vi "StressControl Loop.vi"(6 "Used functions":bool, 8 "error in":errorcluster, 9 "IBM OptoElectroMechanics Configuration":T1={"Parameter Analizer"={"Parameter Analyzer VISA Session"="COM1", "Sweeping Time Parameters"={"Integration Time"=0, "Short Integration Time (s)"=1.0, "Long Integration Time (s)"=0.0, "Wait Time Parameter"=1.0}, "Acquisition Mode"=enum."Sweeping Mode", "Status Polling Time (ms)"=0, "Comment"="Test VI", "SMU 1 - Sweeping"={"Start / Offset"=0.0, "Stop / Ratio"=1.0, "Step \n(linear only)"=0.01, "Compliance"=0.1, "Power \nCompliance"=0.0, "Mode"=0, "Function"=0, "Sweep Mode"=FALSE}, "SMU 2 - Sweeping"={"Start / Offset"=0.0, "Stop / Ratio"=1.0, "Step \n(linear only)"=0.01, "Compliance"=0.1, "Power \nCompliance"=0.0, "Mode"=0, "Function"=0, "Sweep Mode"=FALSE}, "SMU 3 - Sweeping"={"Start / Offset"=0.0, "Stop / Ratio"=1.0, "Step \n(linear only)"=0.01, "Compliance"=0.1, "Power \nCompliance"=0.0, "Mode"=0, "Function"=0, "Sweep Mode"=FALSE}, "SMU 4 - Sweeping"={"Start / Offset"=0.0, "Stop / Ratio"=1.0, "Step \n(linear only)"=0.01, "Compliance"=0.1, "Power \nCompliance"=0.0, "Mode"=0, "Function"=0, "Sweep Mode"=FALSE}, "Sweep Spacing"=0, "Range"=0, "SMU1 - Sampling"={"Source"=10.0, "Compliance"=1e-05, "Mode"=0, "Function"=FALSE}, "SMU2 - Sampling"={"Source"=1.0, "Compliance"=1.0, "Mode"=0, "Function"=FALSE}, "SMU3 - Sampling"={"Source"=10.0, "Compliance"=1e-05, "Mode"=0, "Function"=FALSE}, "SMU4 - Sampling"={"Source"=0.1, "Compliance"=60.0, "Mode"=10, "Function"=FALSE}, "Sampling Time Parameters"={"Initial Interval (s)"=0.1, "Number of Samples"=60, "Total Sampling Time (s)"=10.0, "Hold Time (s)"=0.0, "Sampling Mode"=0, "Sampling Time"=0}, "Stop Condition"={"Enable Delay (s)"=0.0, "Name"="", "Threshold"=0.0, "num. of events"=1, "Event"=0, "Stop Condition Enable"=FALSE}}, "Switching Matrix"={"Switching Matrix VISA Session"="GPIB0::18::INSTR", "Connections"=[{"Connections"=[FALSE, FALSE, FALSE, FALSE, FALSE, FALSE, FALSE, FALSE, FALSE, FALSE, FALSE, FALSE], "Connection Type"=enum."Disconnected"}, {"Connections"=[FALSE, FALSE, FALSE, FALSE, FALSE, FALSE, FALSE, FALSE, FALSE, FALSE, FALSE, FALSE], "Connection Type"=enum."Disconnected"}, {"Connections"=[FALSE, FALSE, FALSE, FALSE, FALSE, FALSE, FALSE, FALSE, FALSE, FALSE, FALSE, FALSE], "Connection Type"=enum."Disconnected"}, {"Connections"=[FALSE, FALSE, FALSE, FALSE, FALSE, FALSE, FALSE, FALSE, FALSE, FALSE, FALSE, FALSE], "Connection Type"=enum."Disconnected"}, {"Connections"=[FALSE, FALSE, FALSE, FALSE, FALSE, FALSE, FALSE, FALSE, FALSE, FALSE, FALSE, FALSE], "Connection Type"=enum."Disconnected"}, {"Connections"=[FALSE, FALSE, FALSE, FALSE, FALSE, FALSE, FALSE, FALSE, FALSE, FALSE, FALSE, FALSE], "Connection Type"=enum."Disconnected"}, {"Connections"=[FALSE, FALSE, FALSE, FALSE, FALSE, FALSE, FALSE, FALSE, FALSE, FALSE, FALSE, FALSE], "Connection Type"=enum."Disconnected"}, {"Connections"=[FALSE, FALSE, FALSE, FALSE, FALSE, FALSE, FALSE, FALSE, FALSE, FALSE, FALSE, FALSE], "Connection Type"=enum."Disconnected"}]}, "Stress Control"={"Stress Control VISA Session"="StrainMotor", "Axis"=0, "Motion"=0, "Destination (°)"=0.0, "Speed (°/s)"=4.0, "Position (°)"=25.0}, "Optical Spectrometer"={"Laser Settings"={"Laser Wavelength"=enum."365 nm", "Neutral Density Filter"=enum."100%"}, "Spectrometer Settings"={"Confocal Hole Size (µm)"=0.0, "Grating"=2, "Detector"=enum."InGaAs Array"}, "Acquisition Settings"={"Acquisition Mode"=enum."Multi-Window", "Spectal Position (nm)"=632.0, "From (nm)"=735.0, "To (nm)"=0.0, "Integration Time (s)"=0.0, "Number of Accumulations"=3, "AutoScanning"=FALSE, "Spike Removal"=FALSE}, "Path"=path "C:/07 - Prizes and Awards/Marie Curie Prize/Reply Editors Final NCOMMS(10).docx"}, "Switches & Mirrors"={"Relay VISA Session"="COM1", "Switches"={"Laser"=FALSE, "Video"=FALSE}, "Delays (ms)"={"Laser"=500, "Video"=1500}}, "Camera"={"Settings"={"Pixel clock"=20, "Frame rate"=30.0, "Exposure time"=33.21525, "Master Gain"=0, "Red Gain"=0, "Green Gain"=0, "Blue Gain"=0, "Auto Gain"=FALSE, "White-balance"=FALSE, "Color Correction"=FALSE}}, "XYZ Stage"={"Connection Settings"={"Tango VISA"="", "Baudrate"=57600, "Show Protocol?"=FALSE}, "Manual Control"={"North"=FALSE, "South"=FALSE, "West"=FALSE, "East"=FALSE, "Up"=FALSE, "Down"=FALSE, "Stop"=FALSE, "XY Step"=0.0, "Z step"=0.0}, "Coordinate Control"={"Motion Mode"=enum."Absolute", "Destination [mm]"=[]}}, "AutoFocus"={"Matching Criteria"={"Minimum Score"=700.0, "Color Score Weight"=700.0, "Minimum Contrast"=50, "Match Mode"=0, "Match Feature Mode"=0, "Subpixel Accuracy"=TRUE, "Color Sensitivity"=1, "Search Strategy"=1}, "Z Scan Parameters"={"Z Range"=1380.0, "Resolution"=5000.0, "Initial Direction"=enum."Up", "Focus Threshold"=0.1, "Ascent Constant"=0.1}, "Displacement"=0.0, "Transformation Matrix"=[]}, "Sava Data"={"Workspace Info"={"Device Name"="ProberHead_Tst_C29K3_7(2)", "Device Info"="ProberHead_Tst_C29", "Path"=path "C:/Users/gio/Desktop/ProbeHeadTest"}, "Instrument Configuration"={"Instrument"=enum."Unknown Instrument", "Configuration"="Test Configuration"}, "Stress Motor Position"=0.0, "Electrical Measurement"={"Sequence"=[], "V1"=[], "V2"=[], "V3"=[], "V4"=[], "I1"=[], "I2"=[], "I3"=[], "I4"=[]}, "Optical Spectrum"={"Intensity"=[], "Wavelength"=[], "Energy"=[], "Raman Shift"=[], "Detector Temperature"=0.0}}, "PlotData"={"Sliders"={"Strain Sequence"=0, "Instrument Sequence"=0}, "Measurement"={"Which Instrument?"=enum."No Plot", "Electrical Measurement"={"Sequence"=[], "V1"=[], "V2"=[], "V3"=[], "V4"=[], "I1"=[], "I2"=[], "I3"=[], "I4"=[]}, "Measurement Mode"=enum."Sweeping Mode", "Optical Spectrum"={"Intensity"=[], "Wavelength"=[], "Energy"=[], "Raman Shift"=[], "Detector Temperature"=0.0}}, "Instrument Steps"=[], "Strain Points"=[]}, "Instrument Sequence"={"Caller VI"=enum."User"}, "Strain Measurement"={"Stress Sequence "={"Max Motor Position"=1380.0, "# Intermediate Points"=5000, "Initial Direction"=enum."Tension"}, "Track?"=FALSE}} {"AutoFocus"."Displacement" scale=1.0..1000.0; "AutoFocus"."Z Scan Parameters"."Focus Threshold" min=0.0 max=1000.0 step=1.0 format="%#_2f"; "AutoFocus"."Z Scan Parameters"."Ascent Constant" min=0.0 max=1000.0 step=1.0 format="%#_2f"; "AutoFocus"."Z Scan Parameters"."Resolution" min=0.0 max=1.0 step=0.01 format="%_2g"; "AutoFocus"."Z Scan Parameters"."Z Range" format="%_3g"; "AutoFocus"."Matching Criteria"."Match Mode" items=["Shift Invariant", "Rotation Invariant"]; "AutoFocus"."Matching Criteria"."Match Feature Mode" items=["Color and Shape", "Color", "Shape"]; "AutoFocus"."Matching Criteria"."Color Sensitivity" items=["Low Sensitivity", "Medium Sensitivity", "High Sensitivity"]; "AutoFocus"."Matching Criteria"."Search Strategy" items=["Conservative", "Balance", "Aggressive", "Very Aggressive"]; "XYZ Stage"."Manual Control"."Z step" scale=0.1..10.0; "XYZ Stage"."Manual Control"."XY Step" scale=0.1..1000.0; "Camera"."Settings"."Blue Gain" min=0 max=100 scale=0.0..100.0; "Camera"."Settings"."Green Gain" min=0 max=100 scale=0.0..100.0; "Camera"."Settings"."Red Gain" min=0 max=100 scale=0.0..100.0; "Camera"."Settings"."Master Gain" min=0 max=100 scale=0.0..100.0; "Camera"."Settings"."Exposure time" min=0.101625 max=159.246375 step=0.101625 scale=0.101625..159.246375 scale format="%#.3g"; "Camera"."Settings"."Frame rate" min=2.7455631699174137 max=6.2675785993528725 step=0.000101625 scale=2.7455631699174137..6.2675785993528725 scale format="%^#_3g"; "Camera"."Settings"."Pixel clock" min=5 max=43 scale=5.0..43.0; "PlotData"."Sliders"."Instrument Sequence" scale=0.0..10.0; "PlotData"."Sliders"."Strain Sequence" scale=0.0..10.0; "Strain Measurement"."Stress Sequence"."# Intermediate Points" max=1390; "Parameter Analizer"."Stop Condition"."Event" items=["Value > Threshold", "Value < Threshold", "| Value | > | Threshold |", "| Value | < | Threshold |"]; "Parameter Analizer"."Stop Condition"."Threshold" format="%^.2e"; "Parameter Analizer"."Stop Condition"."Enable Delay (s)" format="%.1f"; "Parameter Analizer"."Sampling Time Parameters"."Sampling Time" items=["Auto (linear only)", "No Limit", "Set Limit"]; "Parameter Analizer"."Sampling Time Parameters"."Sampling Mode" items=["Linear", "Log10", "Log25", "Log50", "Thinned Out"]; "Parameter Analizer"."Sampling Time Parameters"."Hold Time (s)" format="%.4f"; "Parameter Analizer"."Sampling Time Parameters"."Total Sampling Time (s)" format="%.1f"; "Parameter Analizer"."Sampling Time Parameters"."Initial Interval (s)" format="%^.3e"; "Parameter Analizer"."SMU 4 - Sweeping"."Function" items=["Disabled", "Var 1", "Var 2", "Var 1'", "Constant"]; "Parameter Analizer"."SMU 4 - Sweeping"."Mode" items=["V", "I", "V pulse", "I  pulse", "Common"]; "Parameter Analizer"."SMU 4 - Sweeping"."Power \nCompliance" format="%^.2e"; "Parameter Analizer"."SMU 4 - Sweeping"."Compliance" format="%^.2e"; "Parameter Analizer"."SMU 4 - Sweeping"."Step \n(linear only)" format="%^.4e"; "Parameter Analizer"."SMU 4 - Sweeping"."Stop / Ratio" format="%^.4e"; "Parameter Analizer"."SMU 4 - Sweeping"."Start / Offset" format="%^.4e"; "Parameter Analizer"."SMU 3 - Sweeping"."Function" items=["Disabled", "Var 1", "Var 2", "Var 1'", "Constant"]; "Parameter Analizer"."SMU 3 - Sweeping"."Mode" items=["V", "I", "V pulse", "I  pulse", "Common"]; "Parameter Analizer"."SMU 3 - Sweeping"."Power \nCompliance" format="%^.2e"; "Parameter Analizer"."SMU 3 - Sweeping"."Compliance" format="%^.2e"; "Parameter Analizer"."SMU 3 - Sweeping"."Step \n(linear only)" format="%^.4e"; "Parameter Analizer"."SMU 3 - Sweeping"."Stop / Ratio" format="%^.4e"; "Parameter Analizer"."SMU 3 - Sweeping"."Start / Offset" format="%^.4e"; "Parameter Analizer"."SMU 2 - Sweeping"."Function" items=["Disabled", "Var 1", "Var 2", "Var 1'", "Constant"]; "Parameter Analizer"."SMU 2 - Sweeping"."Mode" items=["V", "I", "V pulse", "I  pulse", "Common"]; "Parameter Analizer"."SMU 2 - Sweeping"."Power \nCompliance" format="%^.2e"; "Parameter Analizer"."SMU 2 - Sweeping"."Compliance" format="%^.2e"; "Parameter Analizer"."SMU 2 - Sweeping"."Step \n(linear only)" format="%^.4e"; "Parameter Analizer"."SMU 2 - Sweeping"."Stop / Ratio" format="%^.4e"; "Parameter Analizer"."SMU 2 - Sweeping"."Start / Offset" format="%^.4e"; "Parameter Analizer"."SMU 1 - Sweeping"."Function" items=["Disabled", "Var 1", "Var 2", "Var 1'", "Constant"]; "Parameter Analizer"."SMU 1 - Sweeping"."Mode" items=["V", "I", "V pulse", "I  pulse", "Common"]; "Parameter Analizer"."SMU 1 - Sweeping"."Power \nCompliance" format="%^.2e"; "Parameter Analizer"."SMU 1 - Sweeping"."Compliance" format="%^.2e"; "Parameter Analizer"."SMU 1 - Sweeping"."Step \n(linear only)" format="%^.4e"; "Parameter Analizer"."SMU 1 - Sweeping"."Stop / Ratio" format="%^.4e"; "Parameter Analizer"."SMU 1 - Sweeping"."Start / Offset" format="%^.4e"; "Parameter Analizer"."Sweeping Time Parameters"."Long Integration Time (s)" scale=0.02..2.0; "Parameter Analizer"."Sweeping Time Parameters"."Short Integration Time (s)" scale=8e-05..0.00192; "Parameter Analizer"."Sweeping Time Parameters"."Integration Time" items=["Short", "Long"]; "Parameter Analizer"."Sweeping Time Parameters"."Wait Time Parameter" format="%.1f"; "Parameter Analizer"."SMU4 - Sampling"."Mode" items=["V", "I", "Common"]; "Parameter Analizer"."SMU4 - Sampling"."Compliance" format="%^.2e"; "Parameter Analizer"."SMU4 - Sampling"."Source" format="%^.3e"; "Parameter Analizer"."SMU3 - Sampling"."Mode" items=["V", "I", "Common"]; "Parameter Analizer"."SMU3 - Sampling"."Compliance" format="%^.2e"; "Parameter Analizer"."SMU3 - Sampling"."Source" format="%^.3e"; "Parameter Analizer"."SMU2 - Sampling"."Mode" items=["V", "I", "Common"]; "Parameter Analizer"."SMU2 - Sampling"."Compliance" format="%^.2e"; "Parameter Analizer"."SMU2 - Sampling"."Source" format="%^.3e"; "Parameter Analizer"."SMU1 - Sampling"."Mode" items=["V", "I", "Common"]; "Parameter Analizer"."SMU1 - Sampling"."Compliance" format="%^.2e"; "Parameter Analizer"."SMU1 - Sampling"."Source" format="%^.3e"; "Parameter Analizer"."Range" items=["auto", "fixed", "limited"]; "Parameter Analizer"."Sweep Spacing" items=["linear", "log 10", "log 25", "log 50"]; "Stress Control"."Axis" min=1 max=3; "Stress Control"."Position (°)" format="%.6g"; "Stress Control"."Speed (°/s)" min=0.0 max=4.0 format="%.6f"; "Stress Control"."Destination (°)" min=-2000000000.0 max=2000000000.0 format="%.6f"; "Stress Control"."Motion" items=["Absolute", "Relative"]; "Optical Spectrometer"."Spectrometer Settings"."Grating" items=["1800 l/mm", "150 l/mm"]}, 10 "Message Queues out":T57, 11 "Notifiers":T44) -> (0 "error out":errorcluster)   [LabVIEW 2014]
uses:
  support/Message Queue/All Message Queues.ctl
  support/Message Queue/Message Cluster.ctl
  support/Notifiers/Notifiers.ctl
  support/Message Handler Loop Notifiers.ctl
  Hardware Control/Parameter Analyzer/Parameter Analyzer Notifiers.ctl
  Hardware Control/Switching Matrix/Switching Matrix Notifiers.ctl
  Hardware Control/Stress Control/StressControl Notifiers.ctl
  Hardware Control/Spectrometer/Spectrometer Notifiers.ctl
  Hardware Control/Switches and Mirrors/SwitchesMirrors Notifiers.ctl
  Hardware Control/Camera/Camera Notifiers.ctl
  Hardware Control/XYZ Stage/XYZ Notifications.ctl
  Hardware Control/Autofocus/Autofocus Notifiers.ctl
  Measurements/Optoelectronic Measurement/Optoelectronic Notifiers.ctl
  Measurements/Save Data/SaveData Notifiers.ctl
  Measurements/Instrument Sequence/Instrument Sequence Notifiers.ctl
  support/Configuration/Configuration.ctl
  Hardware Control/Parameter Analyzer/Parameter Analyzer Config.ctl
  Hardware Control/Parameter Analyzer/Parameter Analyzer Integration Parameters.ctl
  Hardware Control/Parameter Analyzer/Parameter Analyzer SMU Sweeping.ctl
  Hardware Control/Parameter Analyzer/Parameter Analyzer Sweep Spacing.ctl
  Hardware Control/Parameter Analyzer/Parameter Analyzer SMU Range.ctl
  Hardware Control/Parameter Analyzer/Parameter Analyzer SMU Sampling.ctl
  Hardware Control/Parameter Analyzer/Parameter Analyzer Sampling Parameters.ctl
  Hardware Control/Parameter Analyzer/Parameter Analyzer Stop Sampling Conditions.ctl
  Hardware Control/Switching Matrix/Switching Matrix Config.ctl
  Hardware Control/Stress Control/StressControl Config.ctl
  Hardware Control/Spectrometer/Spectrometer Config.ctl
  Hardware Control/Spectrometer/Laser Settings.ctl
  Hardware Control/Spectrometer/Laser.ctl
  Hardware Control/Spectrometer/Filter.ctl
  Hardware Control/Spectrometer/Grating Detector Settings.ctl
  Hardware Control/Spectrometer/Grating.ctl
  Hardware Control/Spectrometer/Detector.ctl
  Hardware Control/Spectrometer/Acquisition Settings.ctl
  Hardware Control/Switches and Mirrors/SwitchesMirrors Config.ctl
  Hardware Control/Switches and Mirrors/SwitchesMirrors Status.ctl
  Hardware Control/Camera/Camera Config.ctl
  Hardware Control/Camera/Camera Settings.ctl
  Hardware Control/XYZ Stage/XYZ Config.ctl
  Hardware Control/XYZ Stage/XYZ Connection Settings.ctl
  Hardware Control/XYZ Stage/XYZ Stage Control.ctl
  Hardware Control/XYZ Stage/XYZ Coordinate Control.ctl
  Hardware Control/Autofocus/AutoFocus Config.ctl
  Hardware Control/Autofocus/ZScan.ctl
  <vilib>/Analysis/Matrix/Datatypes/RealMatrix.ctl
  Measurements/Save Data/SaveData Config.ctl
  Measurements/Save Data/SaveData Workspace Info.ctl
  Measurements/Save Data/SaveData Instrument Configuration.ctl
  Measurements/Instrument Sequence/Instrument List.ctl
  Hardware Control/Spectrometer/Spectral Data.ctl
  Measurements/Plot Data/PlotData Config.ctl
  Measurements/Plot Data/Measurement.ctl
  Measurements/Plot Data/WhichInstrument.ctl
  Hardware Control/Parameter Analyzer/Electrical Data.ctl
  Measurements/Instrument Sequence/Instrument Steps.ctl
  Measurements/Instrument Sequence/Action.ctl
  Measurements/Instrument Sequence/Instrument Sequence Config.ctl
  Measurements/Strain Measurement/Strain Measurement Config.ctl
  Hardware Control/Stress Control/StressControl Functions.ctl
  support/Message Queue/Message Queue.lvlib
  <vilib>/Analysis/Matrix/NI_Matrix.lvlib
panel:
  # "LICENSED MATERIALS – PROPERTY OF IBM\nCopyright IBM Corp. 2016,\nALL RIGHTS RESERVED"
  # "XY"
  # "Z"
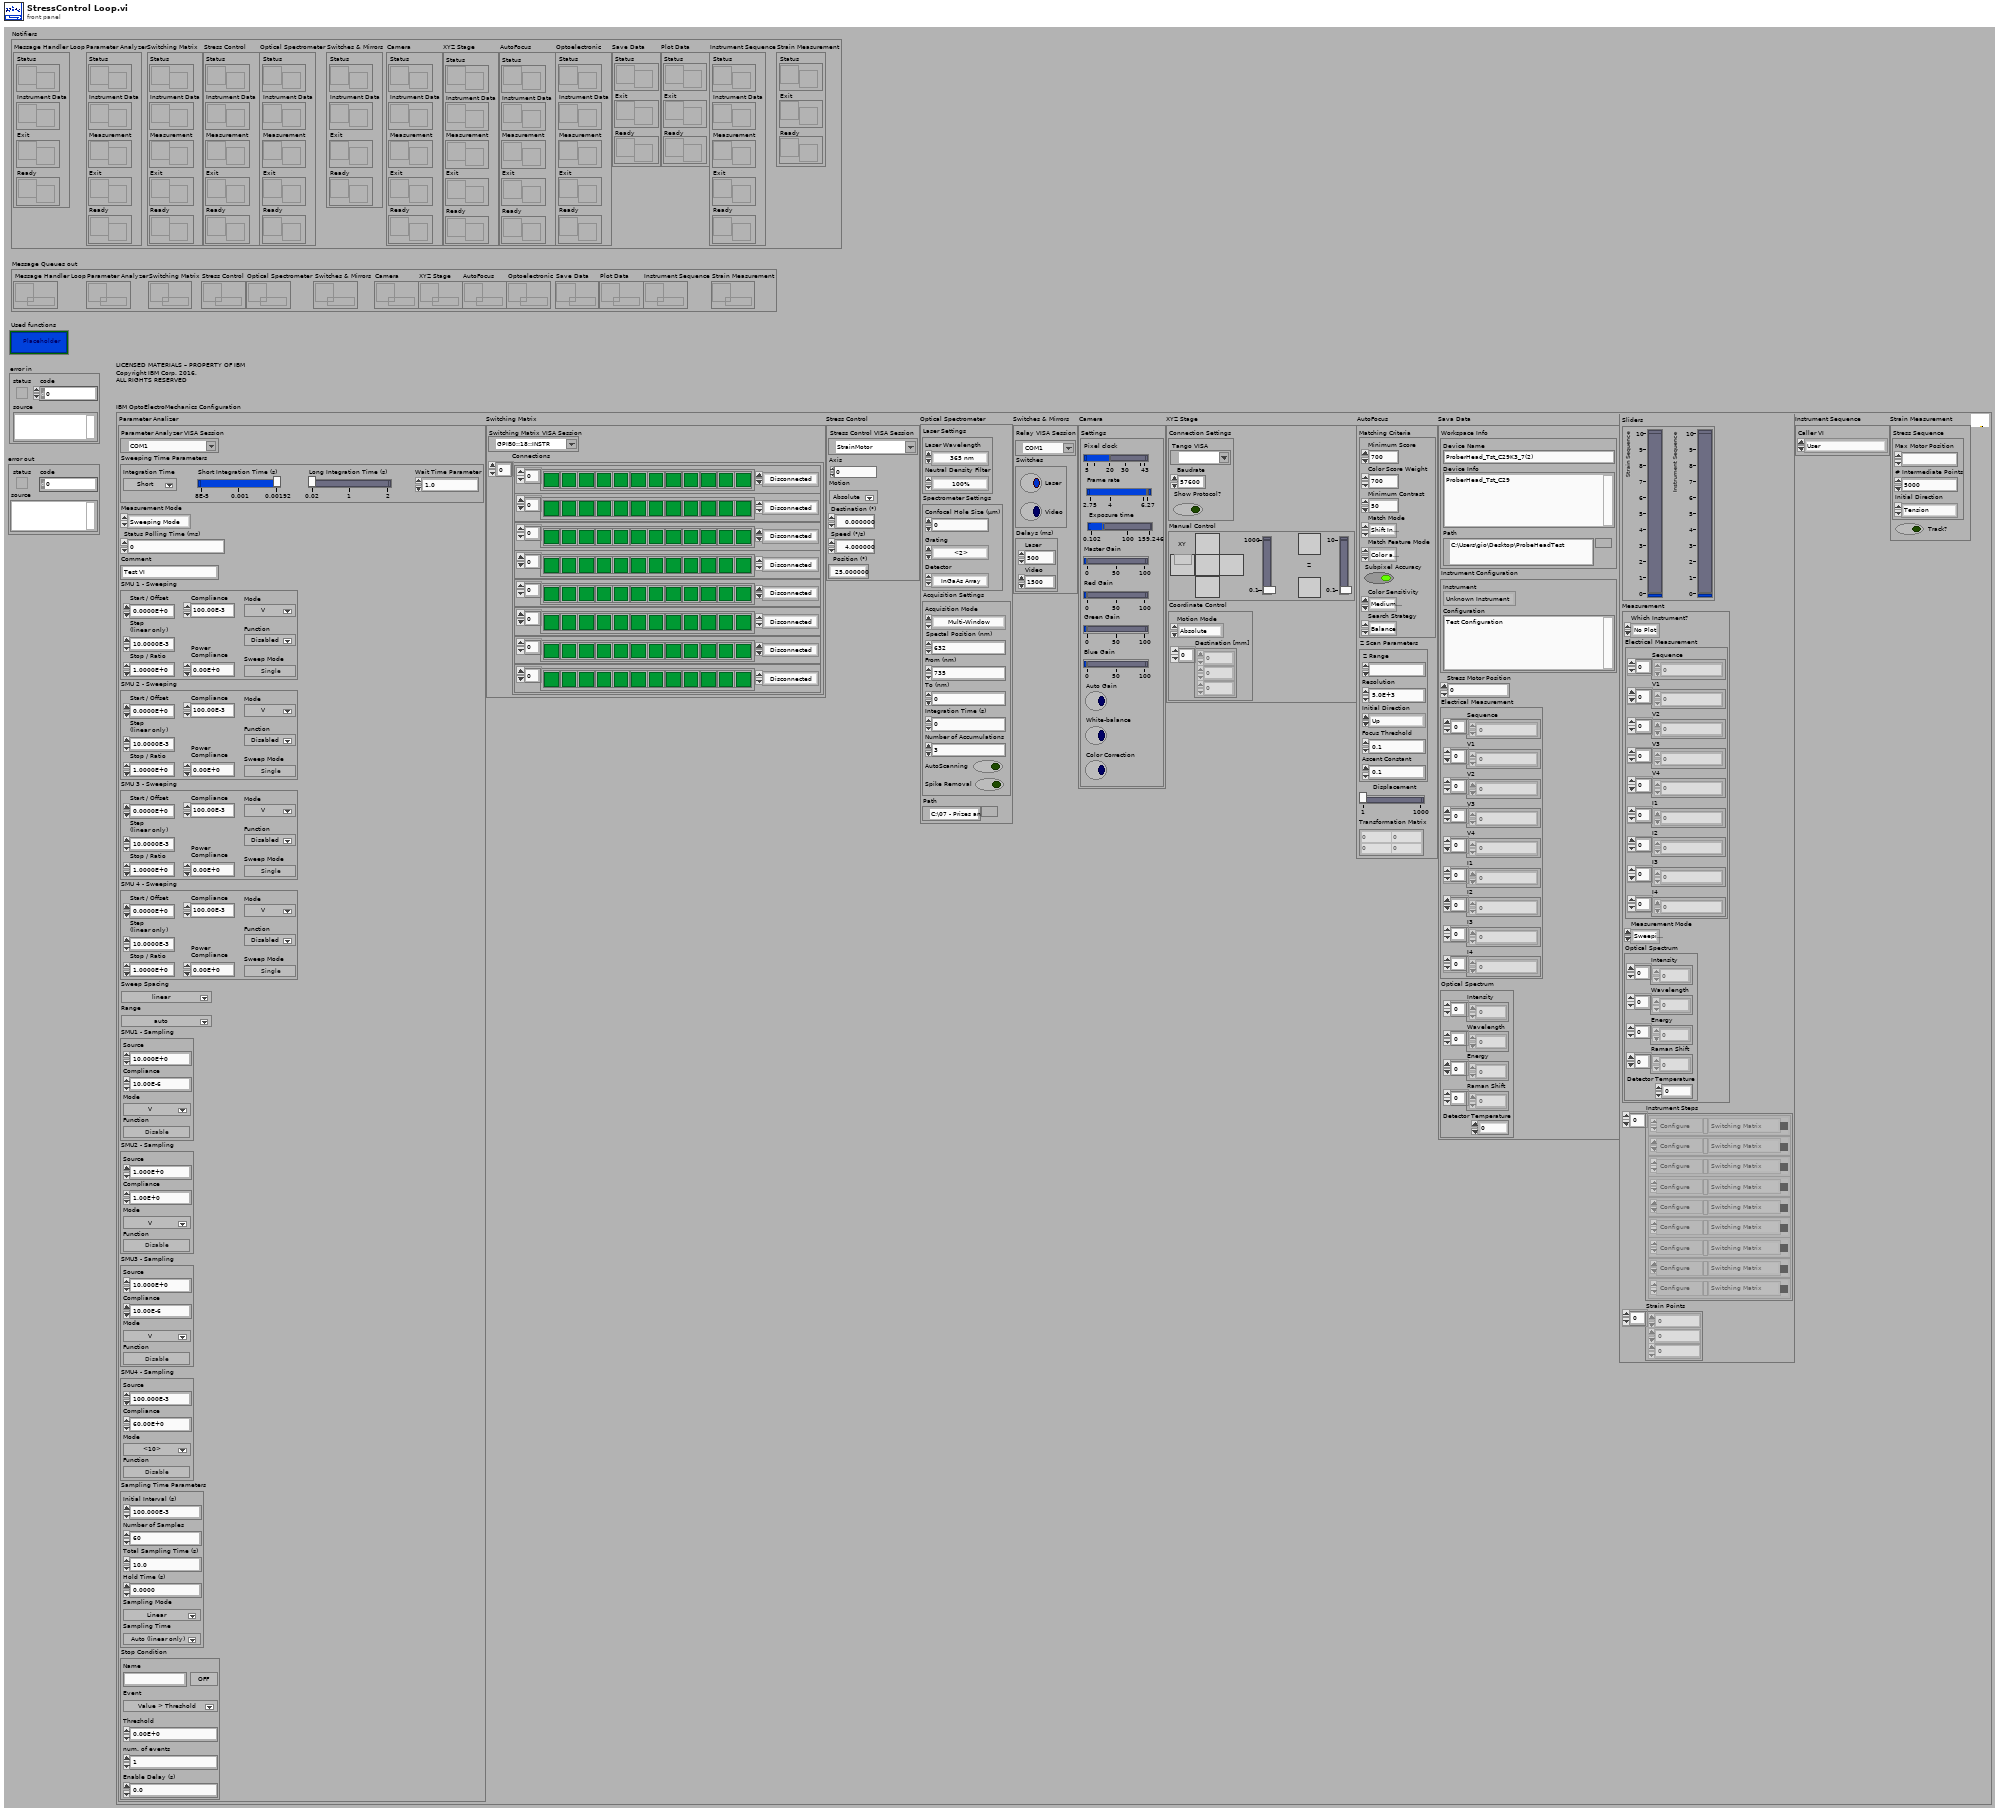
[diagram p1: front panel]
types:
  T1 = typedef "Configuration.ctl" = cluster{"Parameter Analizer":T2, "Switching Matrix":T10, "Stress Control":T11, "Optical Spectrometer":T12, "Switches & Mirrors":T20, "Camera":T22, "XYZ Stage":T24, "AutoFocus":T28, "Sava Data":T31, "PlotData":T36, "Instrument Sequence":T42, "Strain Measurement":T43}
  T2 = typedef "Parameter Analyzer Config.ctl" = cluster{"Parameter Analyzer VISA Session":refnum<visa-resource-name>, "Sweeping Time Parameters":T3, "Acquisition Mode":enum32{"Sweeping Mode", "Sampling Mode"}, "Status Polling Time (ms)":u32, "Comment":string, "SMU 1 - Sweeping":T4, "SMU 2 - Sweeping":T4, "SMU 3 - Sweeping":T4, "SMU 4 - Sweeping":T4, "Sweep Spacing":T5, "Range":T6, "SMU1 - Sampling":T7, "SMU2 - Sampling":T7, "SMU3 - Sampling":T7, "SMU4 - Sampling":T7, "Sampling Time Parameters":T8, "Stop Condition":T9}
  T3 = typedef "Parameter Analyzer Integration Parameters.ctl" = cluster{"Integration Time":u32, "Short Integration Time (s)":dbl, "Long Integration Time (s)":dbl, "Wait Time Parameter":dbl}
  T4 = typedef "Parameter Analyzer SMU Sweeping.ctl" = cluster{"Start / Offset":dbl, "Stop / Ratio":dbl, "Step \n(linear only)":dbl, "Compliance":dbl, "Power \nCompliance":dbl, "Mode":u32, "Function":i32, "Sweep Mode":bool}
  T5 = typedef "Parameter Analyzer Sweep Spacing.ctl" = u16
  T6 = typedef "Parameter Analyzer SMU Range.ctl" = u16
  T7 = typedef "Parameter Analyzer SMU Sampling.ctl" = cluster{"Source":dbl, "Compliance":dbl, "Mode":u32, "Function":bool}
  T8 = typedef "Parameter Analyzer Sampling Parameters.ctl" = cluster{"Initial Interval (s)":dbl, "Number of Samples":i32, "Total Sampling Time (s)":dbl, "Hold Time (s)":dbl, "Sampling Mode":i32, "Sampling Time":i32}
  T9 = typedef "Parameter Analyzer Stop Sampling Conditions.ctl" = cluster{"Enable Delay (s)":dbl, "Name":string, "Threshold":dbl, "num. of events":i32, "Event":i32, "Stop Condition Enable":bool}
  T10 = typedef "Switching Matrix Config.ctl" = cluster{"Switching Matrix VISA Session":refnum<visa-resource-name>, "Connections":cluster{"Connections":bool[], "Connection Type":enum16{"Disconnected", "Make - Break", "Break - Make"}}[]}
  T11 = typedef "StressControl Config.ctl" = cluster{"Stress Control VISA Session":refnum<visa-resource-name>, "Axis":i32, "Motion":u16, "Destination (°)":dbl, "Speed (°/s)":dbl, "Position (°)":dbl}
  T12 = typedef "Spectrometer Config.ctl" = cluster{"Laser Settings":T13, "Spectrometer Settings":T16, "Acquisition Settings":T19, "Path":path}
  T13 = typedef "Laser Settings.ctl" = cluster{"Laser Wavelength":T14, "Neutral Density Filter":T15}
  T14 = typedef "Laser.ctl" = enum16{"633 nm", "784 nm", "532 nm", "365 nm"}
  T15 = typedef "Filter.ctl" = enum16{"100%", "50%", "25%", "10%", "1%", "0.1%", "0.01%"}
  T16 = typedef "Grating Detector Settings.ctl" = cluster{"Confocal Hole Size (µm)":dbl, "Grating":T17, "Detector":T18}
  T17 = typedef "Grating.ctl" = u16
  T18 = typedef "Detector.ctl" = enum16{"InGaAs Array", "Silicon CCD"}
  T19 = typedef "Acquisition Settings.ctl" = cluster{"Acquisition Mode":enum16{"Single Window", "Multi-Window"}, "Spectal Position (nm)":dbl, "From (nm)":dbl, "To (nm)":dbl, "Integration Time (s)":dbl, "Number of Accumulations":i32, "AutoScanning":bool, "Spike Removal":bool}
  T20 = typedef "SwitchesMirrors Config.ctl" = cluster{"Relay VISA Session":refnum<visa-resource-name>, "Switches":T21, "Delays (ms)":cluster{"Laser":u32, "Video":u32}}
  T21 = typedef "SwitchesMirrors Status.ctl" = cluster{"Laser":bool, "Video":bool}
  T22 = typedef "Camera Config.ctl" = cluster{"Settings":T23}
  T23 = typedef "Camera Settings.ctl" = cluster{"Pixel clock":i32, "Frame rate":dbl, "Exposure time":dbl, "Master Gain":i32, "Red Gain":i32, "Green Gain":i32, "Blue Gain":i32, "Auto Gain":bool, "White-balance":bool, "Color Correction":bool}
  T24 = typedef "XYZ Config.ctl" = cluster{"Connection Settings":T25, "Manual Control":T26, "Coordinate Control":T27}
  T25 = typedef "XYZ Connection Settings.ctl" = cluster{"Tango VISA":refnum<visa-resource-name>, "Baudrate":i32, "Show Protocol?":bool}
  T26 = typedef "XYZ Stage Control.ctl" = cluster{"North":bool, "South":bool, "West":bool, "East":bool, "Up":bool, "Down":bool, "Stop":bool, "XY Step":dbl, "Z step":dbl}
  T27 = typedef "XYZ Coordinate Control.ctl" = cluster{"Motion Mode":enum16{"Absolute", "Relative"}, "Destination [mm]":dbl[]}
  T28 = typedef "AutoFocus Config.ctl" = cluster{"Matching Criteria":cluster{"Minimum Score":sgl, "Color Score Weight":sgl, "Minimum Contrast":i32, "Match Mode":u32, "Match Feature Mode":u32, "Subpixel Accuracy":bool, "Color Sensitivity":u32, "Search Strategy":u32}, "Z Scan Parameters":T29, "Displacement":dbl, "Transformation Matrix":T30}
  T29 = typedef "ZScan.ctl" = cluster{"Z Range":ext, "Resolution":dbl, "Initial Direction":enum16{"Up", "Down"}, "Focus Threshold":dbl, "Ascent Constant":dbl}
  T30 = typedef "NI_Matrix.lvlib/RealMatrix.ctl" = dbl[][]
  T31 = typedef "SaveData Config.ctl" = cluster{"Workspace Info":T32, "Instrument Configuration":T33, "Stress Motor Position":dbl, "Electrical Measurement":cluster{"Sequence":dbl[], "V1":dbl[], "V2":dbl[], "V3":dbl[], "V4":dbl[], "I1":dbl[], "I2":dbl[], "I3":dbl[], "I4":dbl[]}, "Optical Spectrum":T35}
  T32 = typedef "SaveData Workspace Info.ctl" = cluster{"Device Name":string, "Device Info":string, "Path":path}
  T33 = typedef "SaveData Instrument Configuration.ctl" = cluster{"Instrument":T34, "Configuration":string}
  T34 = typedef "Instrument List.ctl" = enum32{"Unknown Instrument", "Switching Matrix", "Parameter Analyzer", "Optical Spectrometer", "Optoelectronic", "Autofocus"}
  T35 = typedef "Spectral Data.ctl" = cluster{"Intensity":dbl[], "Wavelength":dbl[], "Energy":dbl[], "Raman Shift":dbl[], "Detector Temperature":dbl}
  T36 = typedef "PlotData Config.ctl" = cluster{"Sliders":cluster{"Strain Sequence":i32, "Instrument Sequence":i32}, "Measurement":T37, "Instrument Steps":T40, "Strain Points":dbl[]}
  T37 = typedef "Measurement.ctl" = cluster{"Which Instrument?":T38, "Electrical Measurement":T39, "Measurement Mode":enum16{"Sweeping Mode", "Sampling Mode"}, "Optical Spectrum":T35}
  T38 = typedef "WhichInstrument.ctl" = enum16{"No Plot", "Spectrometer", "Parameter Analyzer", "Optoelectronic"}
  T39 = typedef "Electrical Data.ctl" = cluster{"Sequence":dbl[], "V1":dbl[], "V2":dbl[], "V3":dbl[], "V4":dbl[], "I1":dbl[], "I2":dbl[], "I3":dbl[], "I4":dbl[]}
  T40 = typedef "Instrument Steps.ctl" = cluster{"Action":T41, "Configuration":variant, "Instrument":T34, "Status":enum8{"False", "True", "Mixed"}}[]
  T41 = typedef "Action.ctl" = enum32{"Configure", "Measure"}
  T42 = typedef "Instrument Sequence Config.ctl" = cluster{"Caller VI":enum16{"User", "Stress Measurement VI"}}
  T43 = typedef "Strain Measurement Config.ctl" = cluster{"Stress Sequence ":cluster{"Max Motor Position":ext, "# Intermediate Points":u32, "Initial Direction":enum16{"Tension", "Compression"}}, "Track?":bool}
  T44 = typedef "Notifiers.ctl" = cluster{"Message Handler Loop":T45, "Parameter Analyzer":T46, "Switching Matrix":T47, "Stress Control":T48, "Optical Spectrometer":T49, "Switches & Mirrors":T50, "Camera":T51, "XYZ Stage":T52, "AutoFocus":T53, "Optoelectronic":T54, "Save Data":T55, "Plot Data":T55, "Instrument Sequence":T56, "Strain Measurement":cluster{"Status":refnum<notifier>, "Exit":refnum<notifier>, "Ready":refnum<notifier>}}
  T45 = typedef "Message Handler Loop Notifiers.ctl" = cluster{"Status":refnum<notifier>, "Instrument Data":refnum<notifier>, "Exit":refnum<notifier>, "Ready":refnum<notifier>}
  T46 = typedef "Parameter Analyzer Notifiers.ctl" = cluster{"Status":refnum<notifier>, "Instrument Data":refnum<notifier>, "Measurement":refnum<notifier>, "Exit":refnum<notifier>, "Ready":refnum<notifier>}
  T47 = typedef "Switching Matrix Notifiers.ctl" = cluster{"Status":refnum<notifier>, "Instrument Data":refnum<notifier>, "Measurement":refnum<notifier>, "Exit":refnum<notifier>, "Ready":refnum<notifier>}
  T48 = typedef "StressControl Notifiers.ctl" = cluster{"Status":refnum<notifier>, "Instrument Data":refnum<notifier>, "Measurement":refnum<notifier>, "Exit":refnum<notifier>, "Ready":refnum<notifier>}
  T49 = typedef "Spectrometer Notifiers.ctl" = cluster{"Status":refnum<notifier>, "Instrument Data":refnum<notifier>, "Measurement":refnum<notifier>, "Exit":refnum<notifier>, "Ready":refnum<notifier>}
  T50 = typedef "SwitchesMirrors Notifiers.ctl" = cluster{"Status":refnum<notifier>, "Instrument Data":refnum<notifier>, "Exit":refnum<notifier>, "Ready":refnum<notifier>}
  T51 = typedef "Camera Notifiers.ctl" = cluster{"Status":refnum<notifier>, "Instrument Data":refnum<notifier>, "Measurement":refnum<notifier>, "Exit":refnum<notifier>, "Ready":refnum<notifier>}
  T52 = typedef "XYZ Notifications.ctl" = cluster{"Status":refnum<notifier>, "Instrument Data":refnum<notifier>, "Measurement":refnum<notifier>, "Exit":refnum<notifier>, "Ready":refnum<notifier>}
  T53 = typedef "Autofocus Notifiers.ctl" = cluster{"Status":refnum<notifier>, "Instrument Data":refnum<notifier>, "Measurement":refnum<notifier>, "Exit":refnum<notifier>, "Ready":refnum<notifier>}
  T54 = typedef "Optoelectronic Notifiers.ctl" = cluster{"Status":refnum<notifier>, "Instrument Data":refnum<notifier>, "Measurement":refnum<notifier>, "Exit":refnum<notifier>, "Ready":refnum<notifier>}
  T55 = typedef "SaveData Notifiers.ctl" = cluster{"Status":refnum<notifier>, "Exit":refnum<notifier>, "Ready":refnum<notifier>}
  T56 = typedef "Instrument Sequence Notifiers.ctl" = cluster{"Status":refnum<notifier>, "Instrument Data":refnum<notifier>, "Measurement":refnum<notifier>, "Exit":refnum<notifier>, "Ready":refnum<notifier>}
  T57 = typedef "Message Queue.lvlib/All Message Queues.ctl" = cluster{"Message Handler Loop":refnum<queue>, "Parameter Analyzer":refnum<queue>, "Switching Matrix":refnum<queue>, "Stress Control":refnum<queue>, "Optical Spectrometer":refnum<queue>, "Switches & Mirrors":refnum<queue>, "Camera":refnum<queue>, "XYZ Stage":refnum<queue>, "AutoFocus":refnum<queue>, "Optoelectronic":refnum<queue>, "Save Data":refnum<queue>, "Plot Data":refnum<queue>, "Instrument Sequence":refnum<queue>, "Strain Measurement":refnum<queue>}
  T58 = typedef "StressControl Data.ctl" = cluster{"Configuration":T11, "Refnums":T59, "Initialization":T60}
  T59 = typedef "StressControl Refnums.ctl" = cluster{"Instrument Status":refnum<vi>, "Position":refnum<vi>, "Mecahnism Motion":refnum<vi>, "Destination":refnum<vi>, "Apply Stress":refnum<vi>, "Stop":refnum<vi>, "Stress Control VISA":refnum<vi>}
  T60 = typedef "StressControl Initialization.ctl" = cluster{"Update Visa Session":bool, "Update Configuration":bool, "Update Refnums":bool, "Get Position":bool}
  T61 = typedef "StressControl Functions.ctl" = enum16{"Connect", "Configure", "Get position", "Move", "Disconnect", "Update Refnums"}
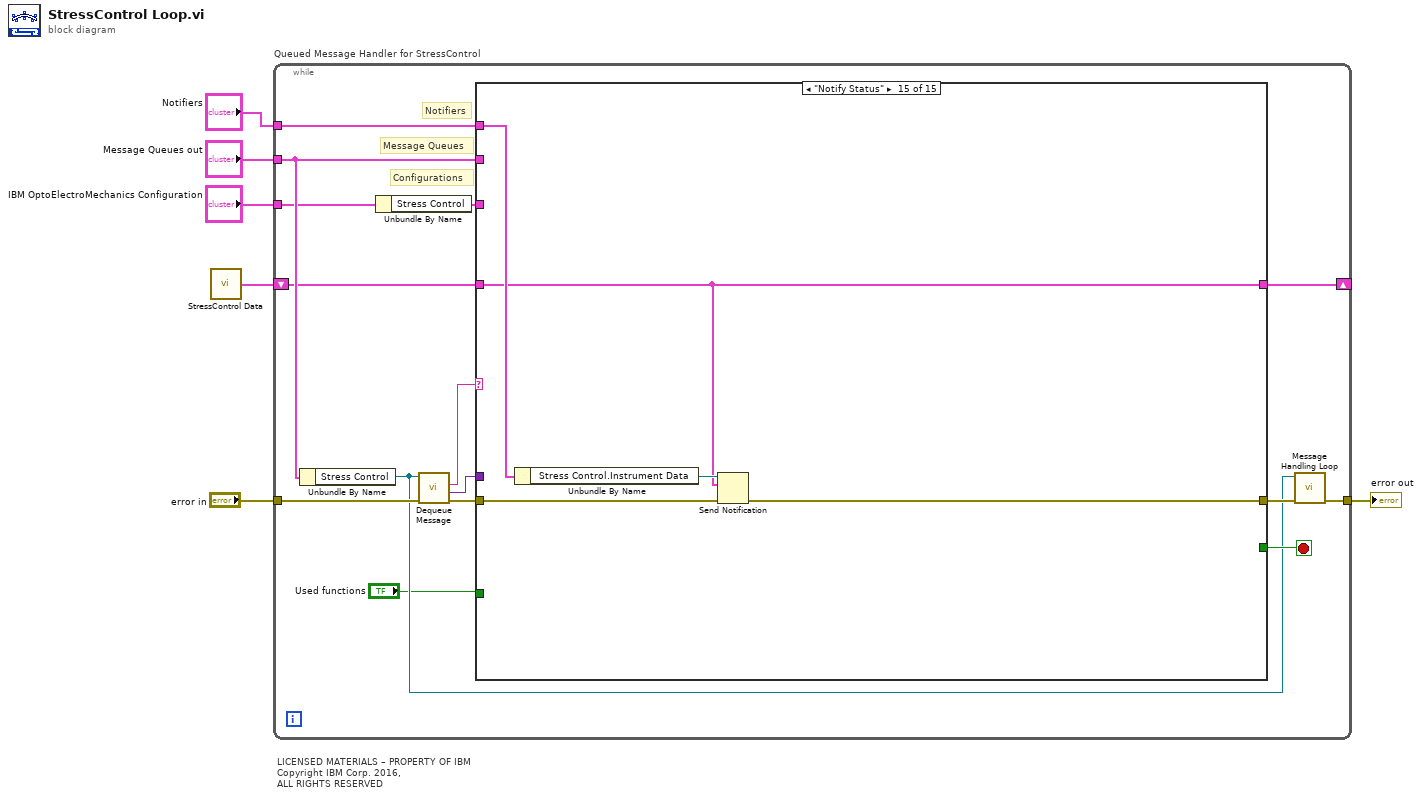
[diagram p0: block diagram]
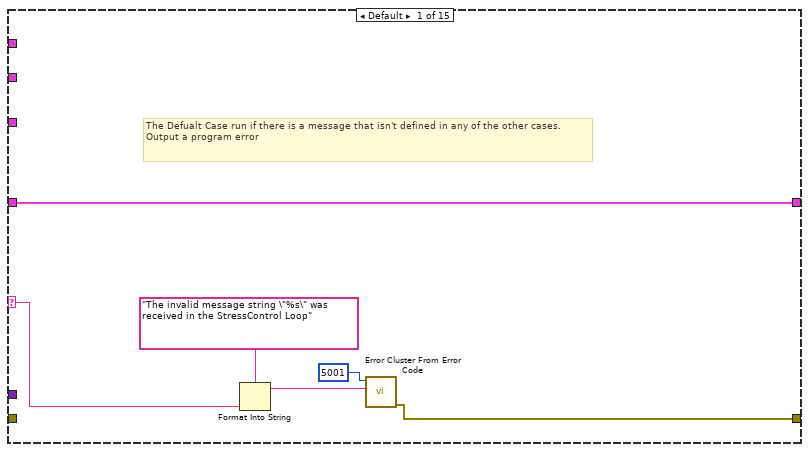
[diagram p2: hidden frame]
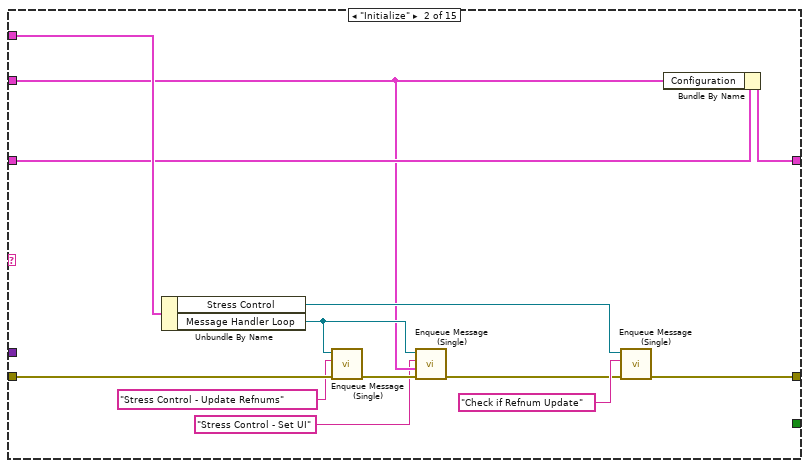
[diagram p3: hidden frame]
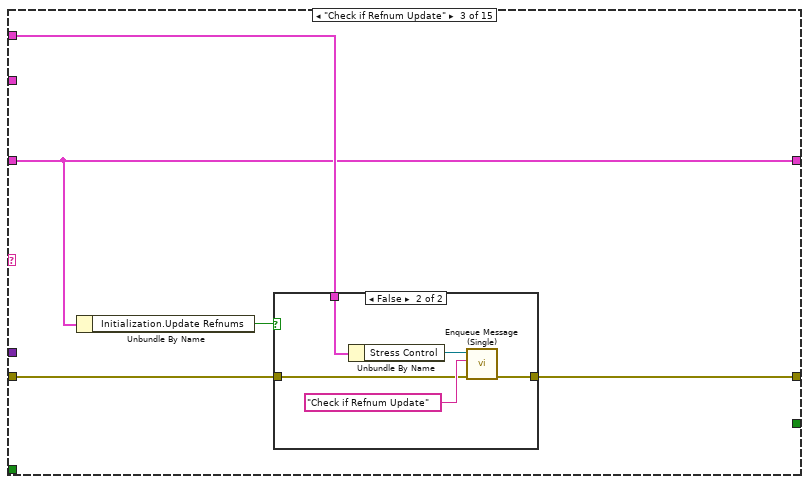
[diagram p4: hidden frame]
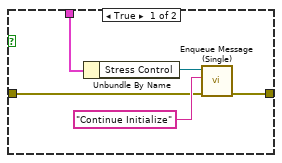
[diagram p5: hidden frame]
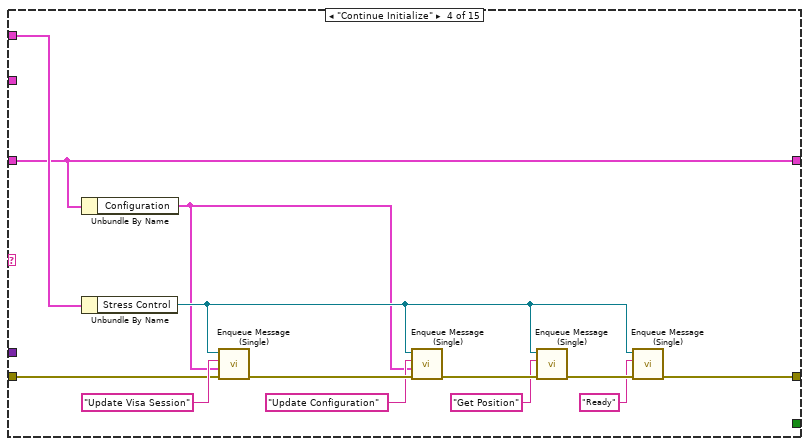
[diagram p6: hidden frame]
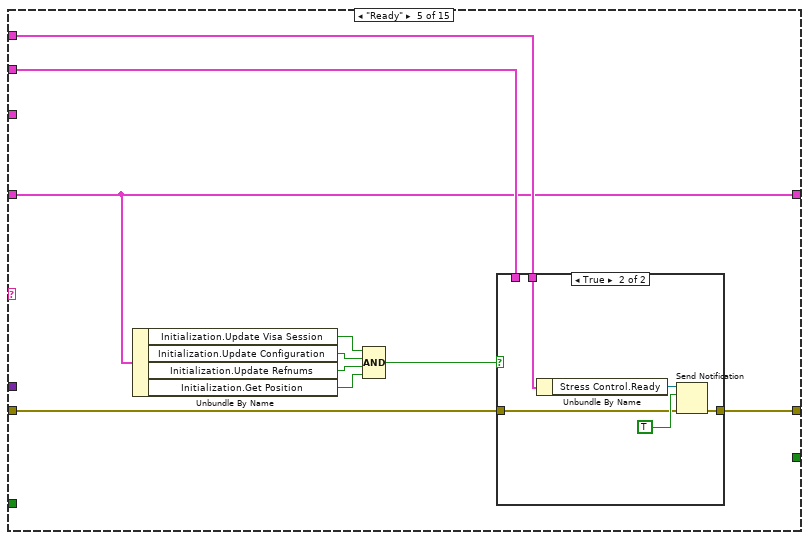
[diagram p7: hidden frame]
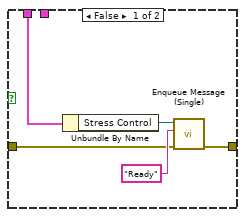
[diagram p8: hidden frame]
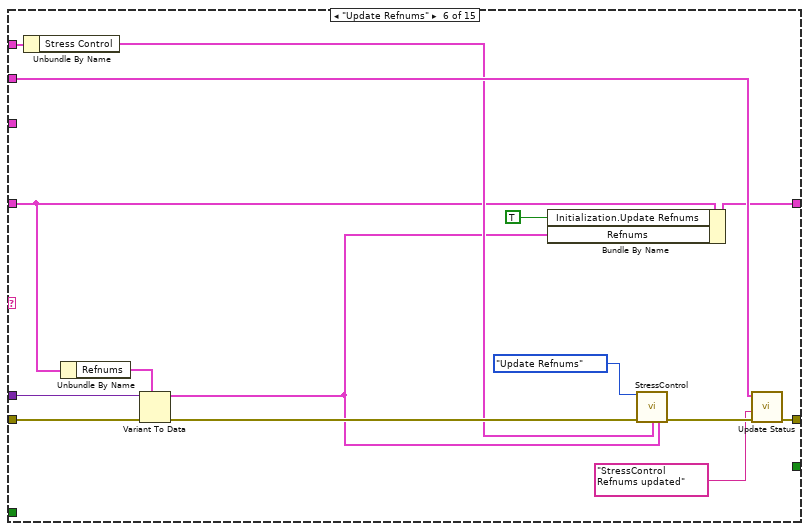
[diagram p9: hidden frame]
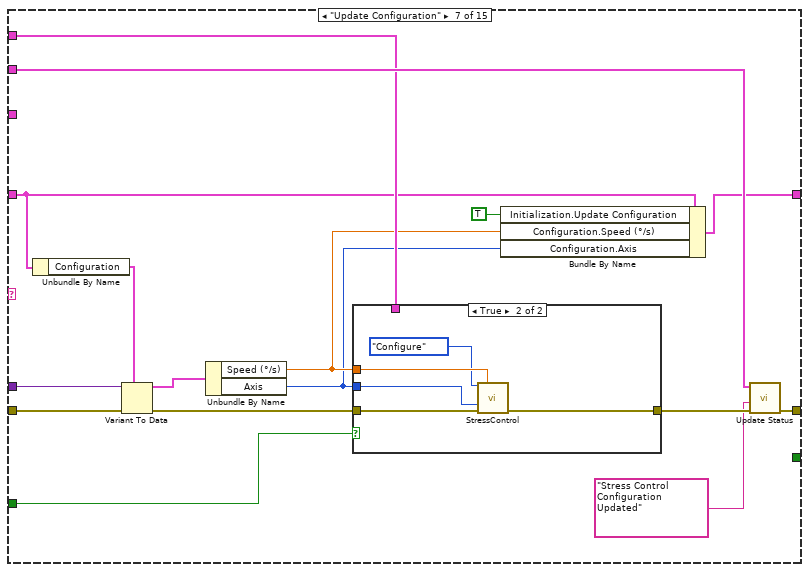
[diagram p10: hidden frame]
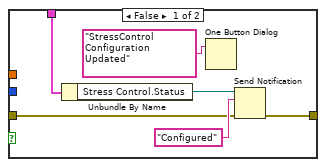
[diagram p11: hidden frame]
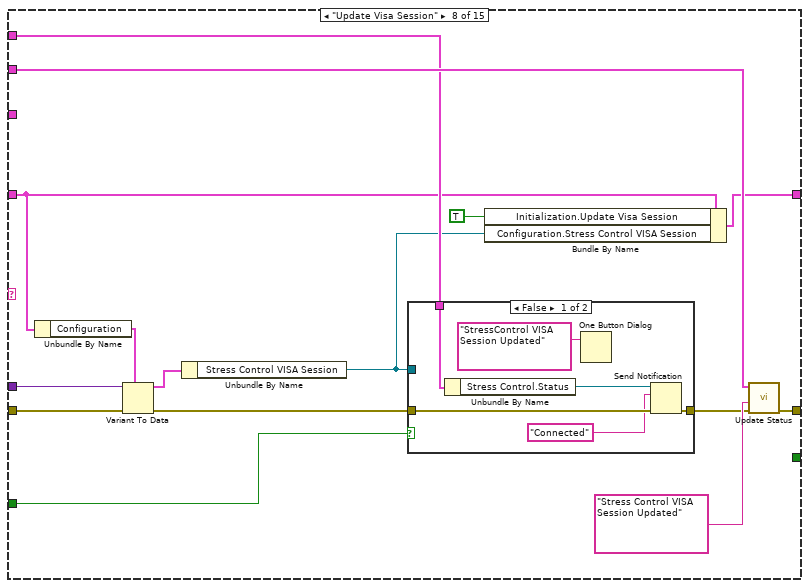
[diagram p12: hidden frame]
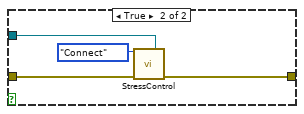
[diagram p13: hidden frame]
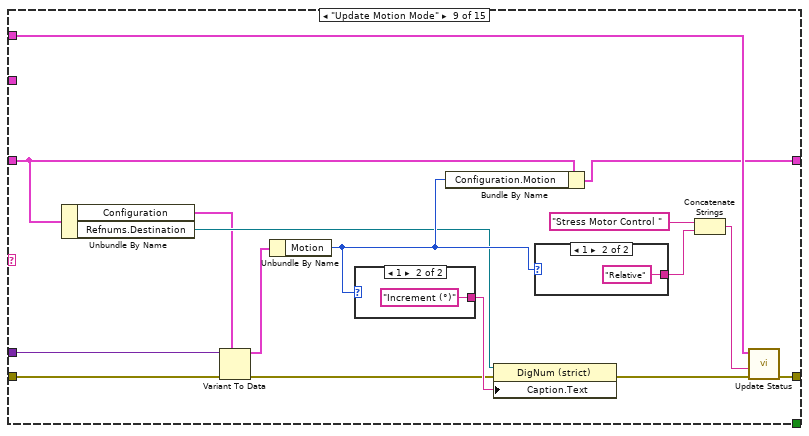
[diagram p14: hidden frame]
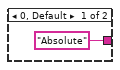
[diagram p15: hidden frame]
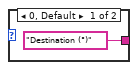
[diagram p16: hidden frame]
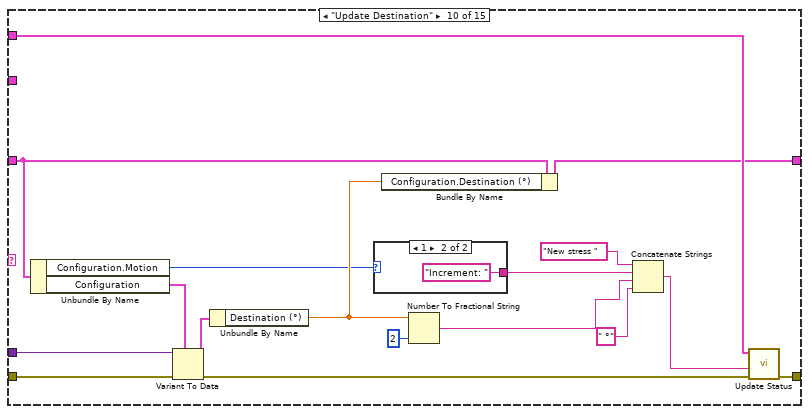
[diagram p17: hidden frame]
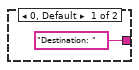
[diagram p18: hidden frame]
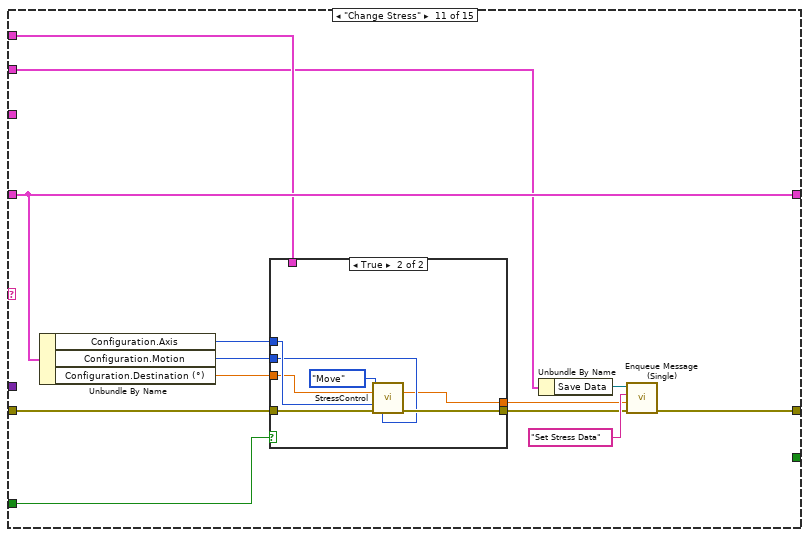
[diagram p19: hidden frame]
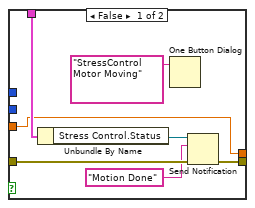
[diagram p20: hidden frame]
diagram:
  # "LICENSED MATERIALS – PROPERTY OF IBM\nCopyright IBM Corp. 2016,\nALL RIGHTS RESERVED"
  n1 = call "StressControl Data.vi"() -> ("Stress Control Data"=w1:T58)
  n2 = while "Queued Message Handler for StressControl" {
    tunnel: "error in" -> [w21]
    tunnel: [w13] -> w2
    tunnel: "Message Queues out" -> [w17]
    tunnel: "Notifiers" -> [w16]
    tunnel: "IBM OptoElectroMechanics Configuration" -> [w11]
    shift-right: [w7] -> _
    shift-left: w1 -> [w8]
    stop <- w15 stop-if-true
    # "Configurations"
    # "Notifiers"
    # "Message Queues"
    n3 = Unbundle By Name(w17) -> ("Stress Control"=w12:refnum<queue>)
    n4 = Unbundle By Name(w11) -> ("Stress Control"=w10:T11)
    n5 = call "Dequeue Message.vi"("error in (no error)"=w21, "Message Queue"=w12) -> ("error out"=w20:errorcluster, "Message Data"=w18:variant, "Message"=w19:string)  [unwired: 7 out]
    n6 = case shown="\"Notify Status\"" w19 {
      selector: w19 -> [w24 _ _ _ _ _ _ _ _ _ _ _ _ _ _]
      tunnel: w20 -> [_ w37 w44 w56 w75 w101 w117 w143 w170 w191 w202 w226 w246 w265 w280]
      tunnel: [w23 w28 w45 w59 w78 w100 w115 w141 w169 w190 w196 w227 w241 w254 w279] -> w14
      tunnel: w18 -> [_ _ _ _ _ w103 w119 w145 w171 w192 _ _ w239 _ _]
      tunnel: w17 -> [_ w40 w43 w67 w77 w97 w112 w140 w168 w189 w198 _ w247 w266 _]
      tunnel: w16 -> [_ _ _ _ w76 w96 w111 w137 _ _ w201 w225 _ w256 w278]
      tunnel: [_ _ _ _ _ _ _ _ _ _ _ _ _ TRUE ("Priority Message? (F)") _] -> w15
      tunnel: w10 -> [_ w30 _ _ _ _ _ _ _ _ _ _ _ _ _]
      tunnel: w8 -> [w22 w39 w42 w57 w74 w91 w105 w132 w157 w178 w203 w223 w238 w262 w276]
      tunnel: "Used functions" -> [_ _ _ _ _ _ w116 w142 _ _ w207 w228 _ w263 _]
      tunnel: [w22 w34 w42 w57 w74 w93 w109 w134 w160 w180 w203 w222 w238 w262 w276] -> w7
      frame Default {
        # "The Defualt Case run if there is a message that isn't defined in any of the other cases.\nOutput a program error"
        n7 = Format Into String(format string="The invalid message string \"%s\" was  received in the StressControl Loop", w24) -> (resulting string=w26:string)  [unwired: 2 in, 1 out]
        n8 = call <vilib>:"Error Cluster From Error Code.vi"("error message (\"\")"=w26, "error code (0)"=5001) -> ("error out"=w23:errorcluster)  [unwired: 2 in, 5 out]
      }
      frame "Initialize" {
        n9 = Unbundle By Name(w40) -> ("Stress Control"=w35:refnum<queue>, "Message Handler Loop"=w32:refnum<queue>)
        n10 = call "Enqueue Message (Single).vi"("error in (no error)"=w37, "Message"="Stress Control - Update Refnums", "Message Queue"=w32) -> ("error out"=w33:errorcluster)  [unwired: 1 in, 7 out]
        n11 = call "Enqueue Message (Single).vi"("error in (no error)"=w33, "Message Data"=w30, "Message"="Stress Control - Set UI", "Message Queue"=w32) -> ("error out"=w31:errorcluster)  [unwired: 7 out]
        n12 = call "Enqueue Message (Single).vi"("error in (no error)"=w31, "Message"="Check if Refnum Update", "Message Queue"=w35) -> ("error out"=w28:errorcluster)  [unwired: 1 in, 7 out]
        n13 = Bundle By Name(cluster=w39, "Configuration"=w30) -> (w34:T58)
      }
      frame "Check if Refnum Update" {
        n14 = Unbundle By Name(w42) -> ("Initialization.Update Refnums"=w41:bool)
        n15 = case shown="False" w41 {
          tunnel: [w48 w53] -> w45
          tunnel: w44 -> [w47 w52]
          tunnel: w43 -> [w46 w51]
          frame True {
            n16 = Unbundle By Name(w46) -> ("Stress Control"=w49:refnum<queue>)
            n17 = call "Enqueue Message (Single).vi"("error in (no error)"=w47, "Message"="Continue Initialize", "Message Queue"=w49) -> ("error out"=w48:errorcluster)  [unwired: 1 in, 7 out]
          }
          frame False {
            n18 = Unbundle By Name(w51) -> ("Stress Control"=w54:refnum<queue>)
            n19 = call "Enqueue Message (Single).vi"("error in (no error)"=w52, "Message"="Check if Refnum Update", "Message Queue"=w54) -> ("error out"=w53:errorcluster)  [unwired: 1 in, 7 out]
          }
        }
      }
      frame "Continue Initialize" {
        n20 = Unbundle By Name(w57) -> ("Configuration"=w58:T11)
        n21 = Unbundle By Name(w67) -> ("Stress Control"=w60:refnum<queue>)
        n22 = call "Enqueue Message (Single).vi"("error in (no error)"=w56, "Message Data"=w58, "Message"="Update Visa Session", "Message Queue"=w60) -> ("error out"=w68:errorcluster)  [unwired: 7 out]
        n23 = call "Enqueue Message (Single).vi"("error in (no error)"=w68, "Message Data"=w58, "Message"="Update Configuration", "Message Queue"=w60) -> ("error out"=w64:errorcluster)  [unwired: 7 out]
        n24 = call "Enqueue Message (Single).vi"("error in (no error)"=w64, "Message"="Get Position", "Message Queue"=w60) -> ("error out"=w62:errorcluster)  [unwired: 1 in, 7 out]
        n25 = call "Enqueue Message (Single).vi"("error in (no error)"=w62, "Message"="Ready", "Message Queue"=w60) -> ("error out"=w59:errorcluster)  [unwired: 1 in, 7 out]
      }
      frame "Ready" {
        n26 = Unbundle By Name(w74) -> ("Initialization.Update Visa Session"=w73:bool, "Initialization.Update Configuration"=w72:bool, "Initialization.Update Refnums"=w71:bool, "Initialization.Get Position"=w70:bool)
        n27 = Compound Arithmetic op=AND(w73, w72, w71, w70) -> (w69:bool)
        n28 = case shown="True" w69 {
          tunnel: [w81 w86] -> w78
          tunnel: w76 -> [_ w85]
          tunnel: w77 -> [w80 _]
          tunnel: w75 -> [w79 w84]
          frame False {
            n29 = Unbundle By Name(w80) -> ("Stress Control"=w83:refnum<queue>)
            n30 = call "Enqueue Message (Single).vi"("error in (no error)"=w79, "Message"="Ready", "Message Queue"=w83) -> ("error out"=w81:errorcluster)  [unwired: 1 in, 7 out]
          }
          frame True {
            n31 = Unbundle By Name(w85) -> ("Stress Control.Ready"=w87:refnum<notifier>)
            n32 = Send Notification(notification=TRUE, notifier=w87, error in (no error)=w84) -> (error out=w86:errorcluster)  [unwired: 1 out]
          }
        }
      }
      frame "Update Refnums" {
        n33 = Unbundle By Name(w96) -> ("Stress Control"=w95:T48)
        n34 = Unbundle By Name(w91) -> ("Refnums"=w90:T59)
        n35 = Variant To Data(error in=w101, type=w90, Variant=w103) -> (data=w89:T59, error out=w102:errorcluster)
        n36 = Bundle By Name(cluster=w91, "Initialization.Update Refnums"=TRUE ("Initialization.Update Visa Session"), "Refnums"=w89) -> (w93:T58)
        n37 = call "StressControl.vi"("Function"=StressControl_Functions."Update Refnums", "error in (no error)"=w102, "StressControl Notifications"=w95, "Motor Refnums"=w89) -> ("error out"=w99:errorcluster)  [unwired: 5 in, 6 out]
        n38 = call "Update Status.vi"("error in"=w99, "String"="StressControl Refnums updated" ("button name (\"OK\")"), "Message Queues out"=w97) -> ("error out"=w100:errorcluster)  [unwired: 8 out]
      }
      frame "Update Configuration" {
        n39 = Unbundle By Name(w105) -> ("Configuration"=w104:T11)
        n40 = Variant To Data(error in=w117, type=w104, Variant=w119) -> (data=w110:T11, error out=w118:errorcluster)
        n41 = Unbundle By Name(w110) -> ("Speed (°/s)"=w107:dbl, "Axis"=w106:i32)
        n42 = case shown="True" w116 {
          tunnel: w118 -> [w122 w130]
          tunnel: [w121 w129] -> w114
          tunnel: w106 -> [_ w128]
          tunnel: w107 -> [_ w127]
          tunnel: w111 -> [w124 _]
          frame False {
            n43 = Unbundle By Name(w124) -> ("Stress Control.Status"=w123:refnum<notifier>)
            n44 = One Button Dialog(message="StressControl Configuration Updated" ("button name (\"OK\")")) -> ()  [unwired: 2 out]
            n45 = Send Notification(notification="Configured", notifier=w123, error in (no error)=w122) -> (error out=w121:errorcluster)  [unwired: 1 out]
          }
          frame True {
            n46 = call "StressControl.vi"("Function"=StressControl_Functions."Configure", "Speed (°/s)"=w127, "Axis"=w128, "error in (no error)"=w130) -> ("error out"=w129:errorcluster)  [unwired: 5 in, 6 out]
          }
        }
        n47 = Bundle By Name(cluster=w105, "Initialization.Update Configuration"=TRUE ("Initialization.Update Visa Session"), "Configuration.Speed (°/s)"=w107, "Configuration.Axis"=w106) -> (w109:T58)
        n48 = call "Update Status.vi"("error in"=w114, "String"="Stress Control Configuration Updated" ("button name (\"OK\")"), "Message Queues out"=w112) -> ("error out"=w115:errorcluster)  [unwired: 8 out]
      }
      frame "Update Visa Session" {
        n49 = Unbundle By Name(w132) -> ("Configuration"=w131:T11)
        n50 = Variant To Data(error in=w143, type=w131, Variant=w145) -> (data=w136:T11, error out=w144:errorcluster)
        n51 = Unbundle By Name(w136) -> ("Stress Control VISA Session"=w133:refnum<visa-resource-name>)
        n52 = case shown="False" w142 {
          tunnel: w144 -> [w151 w155]
          tunnel: [w150 w154] -> w138
          tunnel: w133 -> [_ w153]
          tunnel: w137 -> [w148 _]
          frame False {
            n53 = Unbundle By Name(w148) -> ("Stress Control.Status"=w149:refnum<notifier>)
            n54 = One Button Dialog(message="StressControl VISA Session Updated" ("button name (\"OK\")")) -> ()  [unwired: 2 out]
            n55 = Send Notification(notification="Connected" ("Status"), notifier=w149, error in (no error)=w151) -> (error out=w150:errorcluster)  [unwired: 1 out]
          }
          frame True {
            n56 = call "StressControl.vi"("Function"=StressControl_Functions."Connect", "VISA In"=w153, "error in (no error)"=w155) -> ("error out"=w154:errorcluster)  [unwired: 6 in, 6 out]
          }
        }
        n57 = Bundle By Name(cluster=w132, "Initialization.Update Visa Session"=TRUE, "Configuration.Stress Control VISA Session"=w133) -> (w134:T58)
        n58 = call "Update Status.vi"("error in"=w138, "String"="Stress Control VISA Session Updated" ("button name (\"OK\")"), "Message Queues out"=w140) -> ("error out"=w141:errorcluster)  [unwired: 8 out]
      }
      frame "Update Motion Mode" {
        n59 = Unbundle By Name(w157) -> ("Configuration"=w156:T11, "Refnums.Destination"=w158:refnum<vi>)
        n60 = Variant To Data(error in=w170, type=w156, Variant=w171) -> (data=w167:T11, error out=w162:errorcluster)
        n61 = Unbundle By Name(w167) -> ("Motion"=w159:u16)
        n62 = case shown="1" w159 {
          tunnel: ["Destination (°)" ("Label.Text") "Increment (°)" ("Label.Text")] -> w164
          frame 0, Default {
          }
          frame 1 {
          }
        }
        n63 = Bundle By Name(cluster=w157, "Configuration.Motion"=w159) -> (w160:T58)
        n64 = property on="Property Node" class="DigNum (strict)"(reference=w158, error in=w162, "Caption.Text"=w164) -> (error out=w161:errorcluster)  [unwired: 1 out]
        n65 = case shown="1" w159 {
          tunnel: ["Absolute" ("Label.Text") "Relative" ("Label.Text")] -> w166
          frame 0, Default {
          }
          frame 1 {
          }
        }
        n66 = Concatenate Strings("Stress Motor Control " ("string"), w166) -> (w163:string)
        n67 = call "Update Status.vi"("error in"=w161, "String"=w163, "Message Queues out"=w168) -> ("error out"=w169:errorcluster)  [unwired: 8 out]
      }
      frame "Update Destination" {
        n68 = Unbundle By Name(w178) -> ("Configuration.Motion"=w176:u16, "Configuration"=w177:T11)
        n69 = Variant To Data(error in=w191, type=w177, Variant=w192) -> (data=w183:T11, error out=w182:errorcluster)
        n70 = Unbundle By Name(w183) -> ("Destination (°)"=w179:dbl)
        n71 = case shown="1" w176 {
          tunnel: ["Destination: " ("Label.Text") "Increment: " ("Label.Text")] -> w185
          frame 0, Default {
          }
          frame 1 {
          }
        }
        n72 = Bundle By Name(cluster=w178, "Configuration.Destination (°)"=w179) -> (w180:T58)
        n73 = Number To Fractional String(number=w179, precision (6)=i16 2) -> (F-format string=w188:string)  [unwired: 2 out]
        n74 = Concatenate Strings("New stress " ("string"), w185, w188, " °" ("string")) -> (w181:string)
        n75 = call "Update Status.vi"("error in"=w182, "String"=w181, "Message Queues out"=w189) -> ("error out"=w190:errorcluster)  [unwired: 8 out]
      }
      frame "Change Stress" {
        n76 = Unbundle By Name(w203) -> ("Configuration.Axis"=w206:i32, "Configuration.Motion"=w205:u16, "Configuration.Destination (°)"=w204:dbl)
        n77 = case shown="True" w207 {
          tunnel: w202 -> [w214 w221]
          tunnel: [w213 w220] -> w197
          tunnel: w206 -> [_ w219]
          tunnel: w205 -> [_ w218]
          tunnel: w204 -> [w208 w217]
          tunnel: w201 -> [w212 _]
          tunnel: [w208 w215] -> w195
          frame False {
            n78 = Unbundle By Name(w212) -> ("Stress Control.Status"=w211:refnum<notifier>)
            n79 = One Button Dialog(message="StressControl Motor Moving") -> ()  [unwired: 2 out]
            n80 = Send Notification(notification="Motion Done", notifier=w211, error in (no error)=w214) -> (error out=w213:errorcluster)  [unwired: 1 out]
          }
          frame True {
            n81 = call "StressControl.vi"("Function"=StressControl_Functions."Move", "Destination (°)"=w217, "Axis"=w219, "error in (no error)"=w221, "Motion"=w218) -> ("Position (°)"=w215:dbl, "error out"=w220:errorcluster)  [unwired: 4 in, 5 out]
          }
        }
        n82 = Unbundle By Name(w198) -> ("Save Data"=w199:refnum<queue>)
        n83 = call "Enqueue Message (Single).vi"("error in (no error)"=w197, "Message Data"=w195, "Message"="Set Stress Data", "Message Queue"=w199) -> ("error out"=w196:errorcluster)  [unwired: 7 out]
      }
      frame "Get Position" {
        n84 = case shown="True" w228 {
          tunnel: w226 -> [w234 w237]
          tunnel: [w230 w236] -> w227
          tunnel: w225 -> [w233 _]
          frame False {
            n85 = Unbundle By Name(w233) -> ("Stress Control.Status"=w232:refnum<notifier>)
            n86 = One Button Dialog(message="StressControl Position Updated") -> ()  [unwired: 2 out]
            n87 = Send Notification(notification="Position Acquired", notifier=w232, error in (no error)=w234) -> (error out=w230:errorcluster)  [unwired: 1 out]
          }
          frame True {
            n88 = call "StressControl.vi"("Function"=StressControl_Functions."Get position", "error in (no error)"=w237) -> ("error out"=w236:errorcluster)  [unwired: 7 in, 6 out]
          }
        }
        n89 = Bundle By Name(cluster=w223, "Initialization.Get Position"=TRUE ("Initialization.Update Visa Session")) -> (w222:T58)
      }
      frame "Error" {
        # "Clear Errors to avoid getting stuck \nin repeating this case"
        # "Add here Cases that are handled \nalready by the Message Handler Loop"
        n90 = Variant To Data(error in=w246, type=errorcluster {"status"=FALSE, "code"=0, "source"=""} ("error out"), Variant=w239) -> (data=w245:errorcluster, error out=w244:errorcluster)
        n91 = Merge Errors(w245, w244) -> (w243:errorcluster)
        n92 = Unbundle By Name(w247) -> ("Message Handler Loop"=w249:refnum<queue>)
        n93 = Unbundle By Name(w243) -> ("code"=w240:i32)
        n94 = case shown="Default" w240 {
          tunnel: w249 -> [w253]
          tunnel: w243 -> [w251]
          tunnel: [w250] -> w242
          frame Default {
            n95 = call "Enqueue Message (Single).vi"("Message Data"=w251, "Message"="Error", "Message Queue"=w253) -> ("error out"=w250:errorcluster)  [unwired: 1 in, 7 out]
          }
        }
        n96 = call <vilib>:"Clear Errors.vi"("error in (no error)"=w242) -> ("error out"=w241:errorcluster)  [unwired: 1 in, 5 out]
      }
      frame "Exit" {
        w258 = TRUE ("Priority Message? (F)")
        # "Stip the VI"
        n97 = case shown="True" w263 {
          tunnel: w265 -> [w269 w275]
          tunnel: [w268 w274] -> w264
          tunnel: w256 -> [w272 _]
          frame False {
            n98 = Unbundle By Name(w272) -> ("Stress Control.Status"=w270:refnum<notifier>)
            n99 = Send Notification(notification="Disonnected", notifier=w270, error in (no error)=w269) -> (error out=w268:errorcluster)  [unwired: 1 out]
          }
          frame True {
            n100 = call "StressControl.vi"("Function"=StressControl_Functions."Disconnect", "error in (no error)"=w275) -> ("error out"=w274:errorcluster)  [unwired: 7 in, 6 out]
          }
        }
        n101 = Unbundle By Name(w266) -> ("Stress Control"=w267:refnum<queue>)
        n102 = Unbundle By Name(w256) -> ("Stress Control.Exit"=w257:refnum<notifier>, "Stress Control.Ready"=w260:refnum<notifier>)
        n103 = Release Queue(queue=w267, error in (no error)=w264) -> (error out=w255:errorcluster)  [unwired: 3 out]
        n104 = Send Notification(notification=w258, notifier=w260, error in (no error)=w255) -> (error out=w259:errorcluster)  [unwired: 1 out]
        n105 = Send Notification(notification=w258, notifier=w257, error in (no error)=w259) -> (error out=w254:errorcluster)  [unwired: 1 out]
      }
      frame "Notify Status" {
        n106 = Unbundle By Name(w278) -> ("Stress Control.Instrument Data"=w277:refnum<notifier>)
        n107 = Send Notification(notification=w276, notifier=w277, error in (no error)=w280) -> (error out=w279:errorcluster)  [unwired: 1 out]
      }
    }
    n108 = call "Message Handling Loop.vi"("error in (no error)"=w14, "Message Queue"=w12) -> ("dup error in"=w13:errorcluster)  [unwired: 9 out]
  }
  "error out" <- w2
